vi "Initialize.vi"(6 "optional":variant, 8 "error in (no error)":errorcluster, 11 "TreeNode data":refnum<class "TreeNode.lvclass">) -> (0 "error out":errorcluster, 3 "Node out":refnum<data-value>)   [LabVIEW 2009, in "TreeNode.lvclass"]
uses:
  TreeNode.lvclass
  Node/Node.lvclass
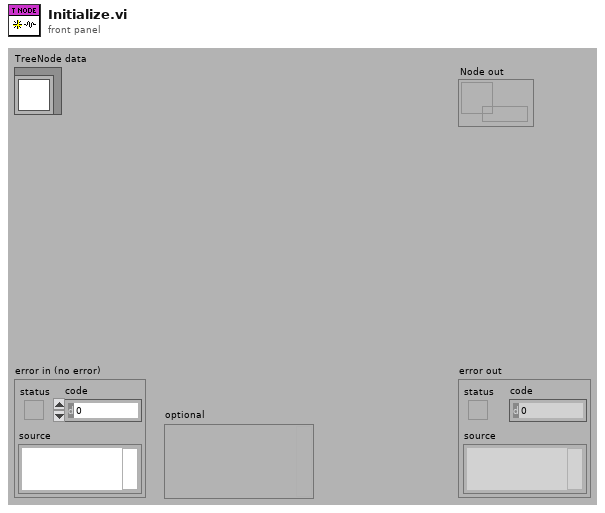
[diagram p1: front panel]
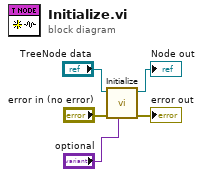
[diagram p0: block diagram]
diagram:
  n1 = call-parent "Initialize.vi"("optional"="optional", "error in (no error)"="error in (no error)", "Node data"="TreeNode data") -> ("error out"=→"error out":errorcluster, "Node out"=→"Node out":refnum<data-value>)  [unwired: 7 in]
